vi "Test Tool Load Unload.vi"() -> ()   [LabVIEW 2011]
uses:
  Shared Components/Gantry Class/Gantry Class.lvclass
  Shared Components/PickupTool Class/PickupTool Class.lvclass
  Shared Components/GrabberTool Class/GrabberTool Class.lvclass
panel:
  out "error out":errorcluster
  in  "Config Folder":path=path "C:/Users/Husker/Desktop/gantry/Config"
  in  "HOME?":bool
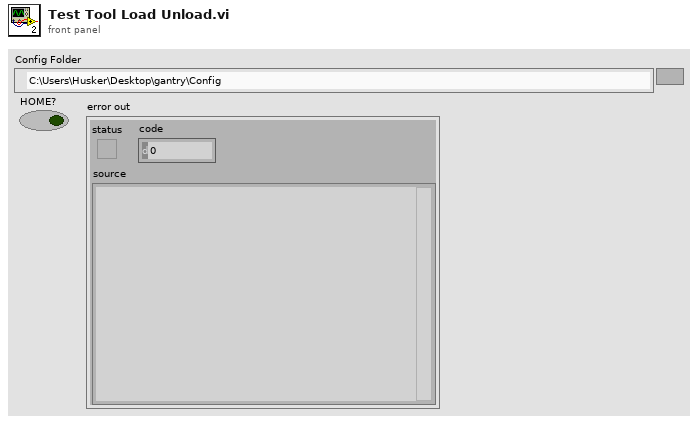
[diagram p1: front panel]
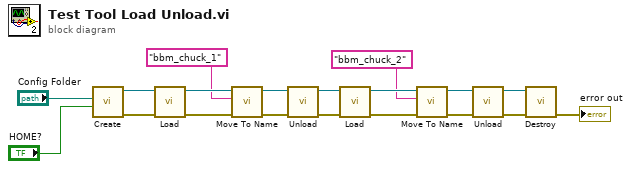
[diagram p0: block diagram]
diagram:
  n1 = call "Create.vi"("HOME?"="HOME?", "Config Folder"="Config Folder") -> ("error out"=w16:errorcluster, "Gantry Class out"=w17:refnum<class "Gantry Class.lvclass">)  [unwired: 8 in]
  n2 = call "Load.vi"("error in (no error)"=w16, "Gantry in"=w17) -> ("error out"=w14:errorcluster, "PickupTool out"=w15:refnum<class "PickupTool Class.lvclass">)  [unwired: 8 in]
  n3 = call "Move To Name.vi"("error in (no error)"=w14, "Destination Name"="bbm_chuck_1", "Gantry in"=w15) -> ("error out"=w11:errorcluster, "Gantry Class out"=w12:refnum<class "PickupTool Class.lvclass">)  [unwired: 7 in]
  n4 = call "Unload.vi"("error in (no error)"=w11, "PickupTool in"=w12) -> ("error out"=w3:errorcluster, "Gantry out"=w4:refnum<class "Gantry Class.lvclass">)  [unwired: 8 in]
  n5 = call "Load.vi"("error in (no error)"=w3, "Gantry In"=w4) -> ("error out"=w8:errorcluster, "Grabber Tool out"=w9:refnum<class "GrabberTool Class.lvclass">)  [unwired: 8 in]
  n6 = call "Move To Name.vi"("error in (no error)"=w8, "Destination Name"="bbm_chuck_2", "Gantry in"=w9) -> ("error out"=w5:errorcluster, "Gantry Class out"=w6:refnum<class "GrabberTool Class.lvclass">)  [unwired: 7 in]
  n7 = call "Unload.vi"("error in (no error)"=w5, "GrabberTool in"=w6) -> ("error out"=w1:errorcluster, "Gantry out"=w2:refnum<class "Gantry Class.lvclass">)  [unwired: 8 in]
  n8 = call "Destroy.vi"("error in (no error)"=w1, "Gantry Class in"=w2) -> ("error out"=→"error out":errorcluster)  [unwired: 9 in]
